vi "写OOC标准.vi"(8 "error in":errorcluster, 9 "threshold":u16, 10 "Base":u16) -> (0 "error out":errorcluster, 2 "return":i32)   [LabVIEW 2016]
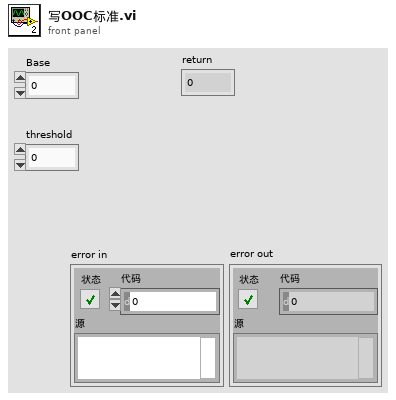
[diagram p1: front panel]
types:
  T1 = cluster{"byCmd":u8, "byLen":u8, "byAddr_h":u8, "byAddr_l":u8}
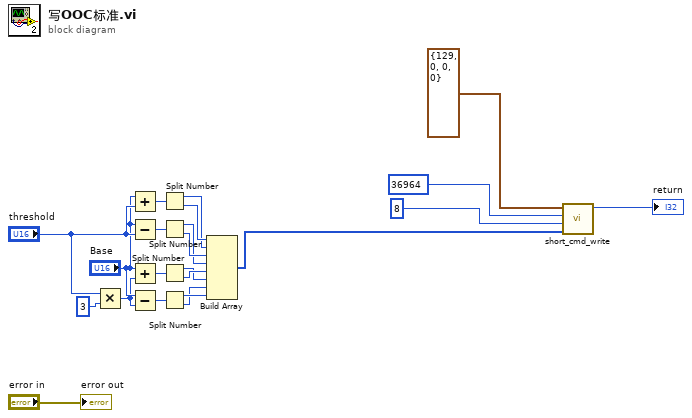
[diagram p0: block diagram]
diagram:
  n1 = Multiply(x="threshold", y=u16 3) -> (x*y=w19:u16)
  n2 = Add(x="Base", y="threshold") -> (x+y=w18:u16)
  n3 = Subtract(x="Base", y="threshold") -> (x-y=w17:u16)
  n4 = Add(x="Base", y=w19) -> (x+y=w16:u16)
  n5 = Subtract(x="Base", y=w19) -> (x-y=w15:u16)
  n6 = Split Number(x=w18) -> (hi(x)=w11:u8, lo(x)=w12:u8)
  n7 = Split Number(x=w17) -> (hi(x)=w9:u8, lo(x)=w10:u8)
  n8 = Split Number(x=w16) -> (hi(x)=w7:u8, lo(x)=w8:u8)
  n9 = Split Number(x=w15) -> (hi(x)=w6:u8, lo(x)=w5:u8)
  n10 = Build Array(w12, w11, w10, w9, w8, w7, w5, w6) -> (w3:u8[])
  n11 = call "short_cmd_write.vi"("data"=w3, "dwLen"=u16 8, "dwAddr"=u16 36964, "cmd_short_header_t"=T1 {"byCmd"=129, "byLen"=0, "byAddr_h"=0, "byAddr_l"=0}) -> ("return"=→"return":i32)  [unwired: 7 in]
  "error out" <- "error in"
